vi "System Explorer - Add PPL content to System Explorer library.vi"(8 "error in (no error)":errorcluster, 9 "Extra Page Names":string[](array[string]), 10 "Project Root":path, 11 "CD Wizard - Internal Data":T1) -> (0 "error out":errorcluster, 1 "Extra Page VIs":path[](array[path]), 2 "System Explorer Main VI":path, 3 "Load Help File VI":path)   [LabVIEW 2019, in "NIVS_Consolidated_CDW_MetaDataObj.lvclass"]
doc: "Add all virtual folders and VIs to the System Explorer library."
uses:
  Internal data.ctl
  CD System Explorer lvlib.ctl
  Add Item - Type.ctl
  CD System Explorer lvlib.vi
  NIVS_Consolidated_CDW_MetaDataObj.lvclass
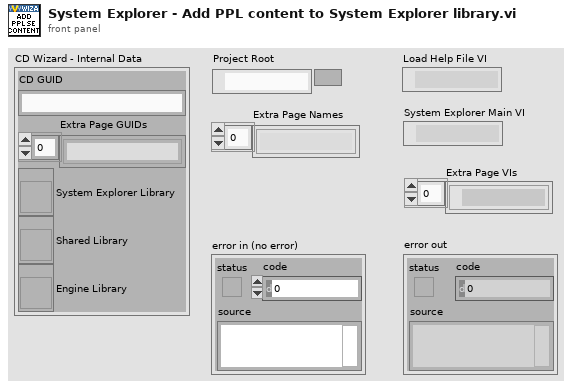
[diagram p1: front panel]
types:
  T1 = typedef "NIVS_Consolidated_CDW_MetaDataObj.lvclass/Internal data.ctl" = cluster{"CD GUID":string, "Extra Page GUIDs":string[], "System Explorer Library":refnum<vi>, "Shared Library":refnum<vi>, "Engine Library":refnum<vi>}
  T2 = typedef "NIVS_Consolidated_CDW_MetaDataObj.lvclass/CD System Explorer lvlib.ctl" = enum16{"LibraryFileName", "LibraryFolderName", "System Explorer.FolderName", "System Explorer.Dynamically Called.FolderName", "System Explorer.Dynamically Called.Extra Pages.FolderName", "System Explorer.Dynamically Called.Extra Pages.TemplatePathAndName", "System Explorer.Dynamically Called.Main Page.VIName", "System Explorer.Dynamically Called.Main Page.TemplatePathAndName", "System Explorer.Dynamically Called.Initialization VI.VIName", "System Explorer.Dynamically Called.Initialization VI.TemplatePathAndName", "System Explorer.SubVI.FolderName", "System Explorer.Types.FolderName", "System Explorer.ActionVIOnCompile.VIName", "System Explorer.ExportConfigRTM.VIName", "System Explorer.LoadHelpFile.VIName", "System Explorer.SetRTDriverVIsFilePaths.VIName", "System Explorer.ClearRTDriverVIs.VIName"}
  T3 = typedef "NIVS_Consolidated_CDW_MetaDataObj.lvclass/Add Item - Type.ctl" = string
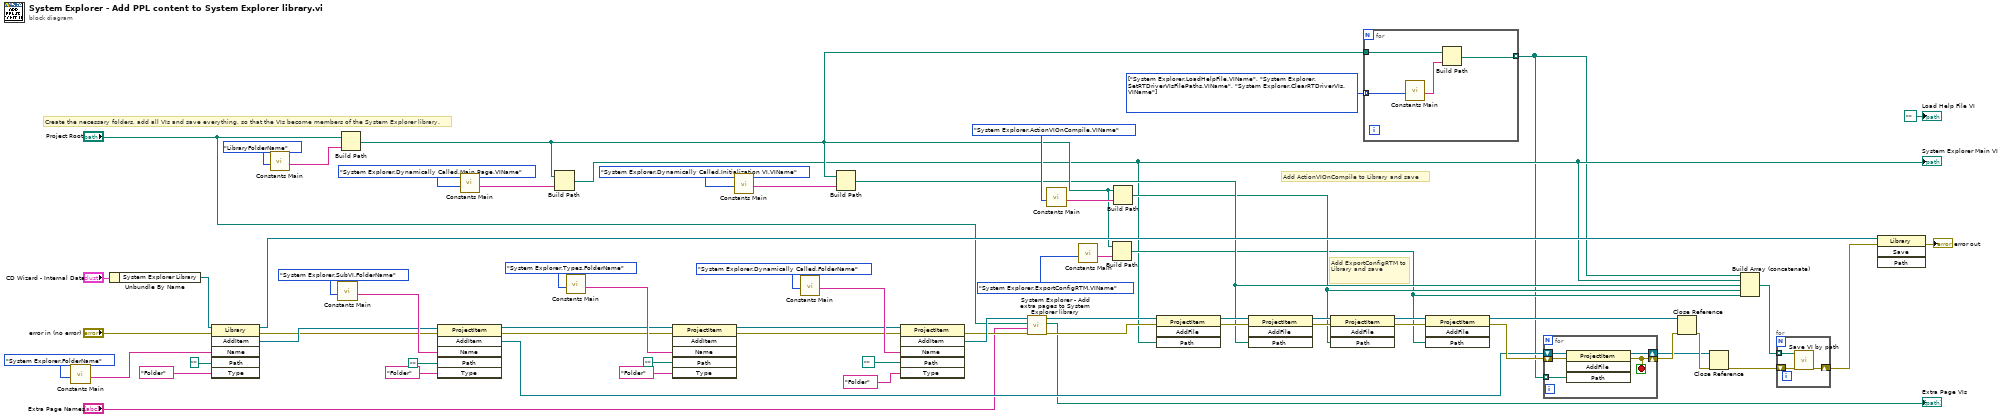
[diagram p0: block diagram]
diagram:
  w11 = T2[] [enum."System Explorer.LoadHelpFile.VIName", enum."System Explorer.SetRTDriverVIsFilePaths.VIName", enum."System Explorer.ClearRTDriverVIs.VIName"] items=["LibraryFileName", "LibraryFolderName", "System Explorer.FolderName", "System Explorer.Dynamically Called.FolderName", "System Explorer.Dynamically Called.Extra Pages.FolderName", "System Explorer.Dynamically Called.Extra Pages.TemplatePathAndName", "System Explorer.Dynamically Called.Main Page.VIName", "System Explorer.Dynamically Called.Main Page.TemplatePathAndName", "System Explorer.Dynamically Called.Initialization VI.VIName", "System Explorer.Dynamically Called.Initialization VI.TemplatePathAndName", "System Explorer.SubVI.FolderName", "System Explorer.Types.FolderName", "System Explorer.ActionVIOnCompile.VIName", "System Explorer.ExportConfigRTM.VIName", "System Explorer.LoadHelpFile.VIName", "System Explorer.SetRTDriverVIsFilePaths.VIName", "System Explorer.ClearRTDriverVIs.VIName"]
  # "Create the necessary folders, add all VIs and save everything, so that the VIs become members of the System Explorer library."
  # "Add ExportConfigRTM to Library and save"
  # "Add ActionVIOnCompile to Library and save"
  n1 = call-poly "Constants Main.vi"("Action"=CD_System_Explorer_lvlib."System Explorer.FolderName") -> ("Output"=w62:string)  [unwired: 10 in]
  n2 = Unbundle By Name("CD Wizard - Internal Data") -> ("System Explorer Library"=w39:refnum<vi>)
  n3 = invoke class="Library" method="AddItem"(reference=w39, error in="error in (no error)", "Name"=w62, "Path"=path "", "Type"=T3 "Folder" ("Add Item - Type")) -> (reference out=w41:refnum<vi>, error out=w18:errorcluster, "AddItem"=w40:refnum<vi>)  [unwired: 1 in, 3 out]
  n4 = call-poly "Constants Main.vi"("Action"=CD_System_Explorer_lvlib."LibraryFolderName") -> ("Output"=w34:string)  [unwired: 10 in]
  n5 = call-poly "Constants Main.vi"("Action"=CD_System_Explorer_lvlib."System Explorer.SubVI.FolderName") -> ("Output"=w56:string)  [unwired: 10 in]
  n6 = Build Path(base path="Project Root", name or relative path=w34) -> (appended path=w10:path)
  n7 = invoke class="ProjectItem" method="AddItem"(reference=w40, error in=w18, "Name"=w56, "Path"=path "", "Type"=T3 "Folder" ("Add Item - Type")) -> (reference out=w43:refnum<vi>, error out=w17:errorcluster, "AddItem"=w20:refnum<vi>)  [unwired: 1 in, 3 out]
  n8 = call-poly "Constants Main.vi"("Action"=CD_System_Explorer_lvlib."System Explorer.Dynamically Called.Main Page.VIName") -> ("Output"=w60:string)  [unwired: 10 in]
  n9 = Build Path(base path=w10, name or relative path=w60) -> (appended path=w2:path)
  "System Explorer Main VI" <- w2
  n10 = call-poly "Constants Main.vi"("Action"=CD_System_Explorer_lvlib."System Explorer.Types.FolderName") -> ("Output"=w51:string)  [unwired: 10 in]
  n11 = invoke class="ProjectItem" method="AddItem"(reference=w43, error in=w17, "Name"=w51, "Path"=path "", "Type"=T3 "Folder" ("Add Item - Type")) -> (reference out=w42:refnum<vi>, error out=w16:errorcluster)  [unwired: 1 in, 4 out]
  n12 = call-poly "Constants Main.vi"("Action"=CD_System_Explorer_lvlib."System Explorer.Dynamically Called.Initialization VI.VIName") -> ("Output"=w59:string)  [unwired: 10 in]
  n13 = call-poly "Constants Main.vi"("Action"=CD_System_Explorer_lvlib."System Explorer.Dynamically Called.FolderName") -> ("Output"=w46:string)  [unwired: 10 in]
  n14 = Build Path(base path=w10, name or relative path=w59) -> (appended path=w7:path)
  n15 = invoke class="ProjectItem" method="AddItem"(reference=w42, error in=w16, "Name"=w46, "Path"=path "", "Type"=T3 "Folder" ("Add Item - Type")) -> (error out=w36:errorcluster, "AddItem"=w38:refnum<vi>)  [unwired: 1 in, 4 out]
  n16 = call "System Explorer - Add extra pages to System Explorer library.vi"("error in (no error)"=w36, "Extra Page Names"="Extra Page Names", "Project Root"="Project Root", "ProjectItem in"=w38) -> ("error out"=w15:errorcluster, "Extra Page VIs"=→"Extra Page VIs":path[], "ProjectItem out"=w37:refnum<vi>)  [unwired: 5 in]
  n17 = call-poly "Constants Main.vi"("Action"=CD_System_Explorer_lvlib."System Explorer.ActionVIOnCompile.VIName") -> ("Output"=w30:string)  [unwired: 10 in]
  n18 = call-poly "Constants Main.vi"("Action"=CD_System_Explorer_lvlib."System Explorer.ExportConfigRTM.VIName") -> ("Output"=w25:string)  [unwired: 10 in]
  n19 = Build Path(base path=w10, name or relative path=w25) -> (appended path=w5:path)
  n20 = Build Path(base path=w10, name or relative path=w30) -> (appended path=w6:path)
  n21 = invoke class="ProjectItem" method="AddFile"(reference=w37, error in=w15, "Path"=w2) -> (reference out=w44:refnum<vi>, error out=w45:errorcluster)  [unwired: 1 in, 2 out]
  n22 = invoke class="ProjectItem" method="AddFile"(reference=w44, error in=w45, "Path"=w7) -> (reference out=w33:refnum<vi>, error out=w32:errorcluster)  [unwired: 1 in, 2 out]
  n23 = invoke class="ProjectItem" method="AddFile"(reference=w33, error in=w32, "Path"=w6) -> (reference out=w29:refnum<vi>, error out=w23:errorcluster)  [unwired: 1 in, 2 out]
  n24 = for {
    tunnel: w11 -> [w71] mode=indexing
    tunnel: w10 -> [w69]
    tunnel: [w68] -> w1 mode=indexing
    n25 = call-poly "Constants Main.vi"("Action"=w71) -> ("Output"=w70:string)  [unwired: 10 in]
    n26 = Build Path(base path=w69, name or relative path=w70) -> (appended path=w68:path)
  }
  n27 = invoke class="ProjectItem" method="AddFile"(reference=w29, error in=w23, "Path"=w5) -> (reference out=w22:refnum<vi>, error out=w28:errorcluster)  [unwired: 1 in, 2 out]
  n28 = for {
    shift-right: [w72] -> w24
    shift-left: w28 -> [w76]
    shift-right: [w75] -> w21
    shift-left: w20 -> [w74]
    tunnel: w1 -> [w73] mode=indexing
    stop <- w72 stop-if-true
    n29 = invoke class="ProjectItem" method="AddFile"(reference=w74, error in=w76, "Path"=w73) -> (reference out=w75:refnum<vi>, error out=w72:errorcluster)  [unwired: 1 in, 2 out]
  }
  n30 = Close Reference(reference=w22, error in (no error)=w24) -> (error out=w27:errorcluster)
  n31 = Close Reference(reference=w21, error in (no error)=w27) -> (error out=w3:errorcluster)
  n32 = Build Array (concatenate)(w1, w2, w7, w6, w5) -> (w4:path[])
  n33 = for {
    tunnel: w4 -> [w79] mode=indexing
    shift-right: [w77] -> w8
    shift-left: w3 -> [w78]
    n34 = call "Save VI by path.vi"("error in (no error)"=w78, "VI path"=w79) -> ("error out"=w77:errorcluster)  [unwired: 9 in]
  }
  n35 = invoke class="Library" method="Save"(reference=w41, error in=w8) -> (error out=→"error out":errorcluster)  [unwired: 2 in, 3 out]
  "Load Help File VI" <- path "" ("Load Help File VI")
